vi "Simple UDP - Receiver.vi"() -> ()   [LabVIEW 2014]
doc: "The UDP protocol differs from TCP in that there is no error-checking with the packets of information that are sent, and thus no guarantee whatsoever that an intended recipient will actually receive a given piece of data.\n\nUDP does offer the ability to \"broadcast\" data across a network--simply specify an IP Address of all ones (255.255.255.255) to attempt to broadcast information network-wide. Keep in mind that routers and other network hardware will generally refuse to forward the broadcast beyond certain points, so the extent of the broadcast will in practice be limited."
panel:
  out "Waveform Chart":u8(graph)
  in  "Stop":bool
  # "Overview: Demonstrates the use of the UDP functions to receive data over a UDP connection.\nInstructions:\n1. Ensure Simple UDP - Sender.vi is already running.\n2. Run the VI.\n3. Click Stop to stop the VI."
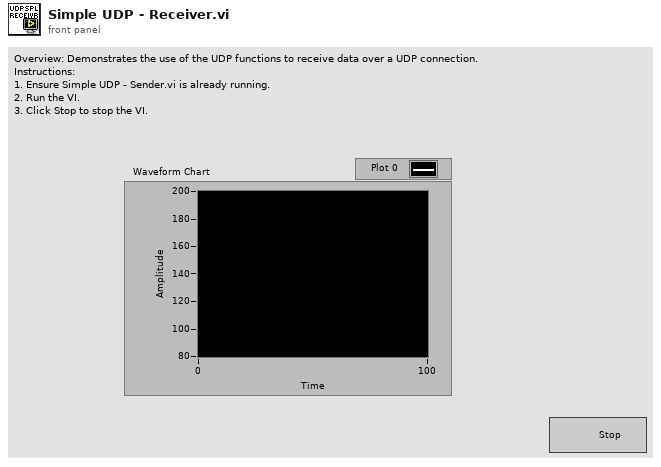
[diagram p1: front panel]
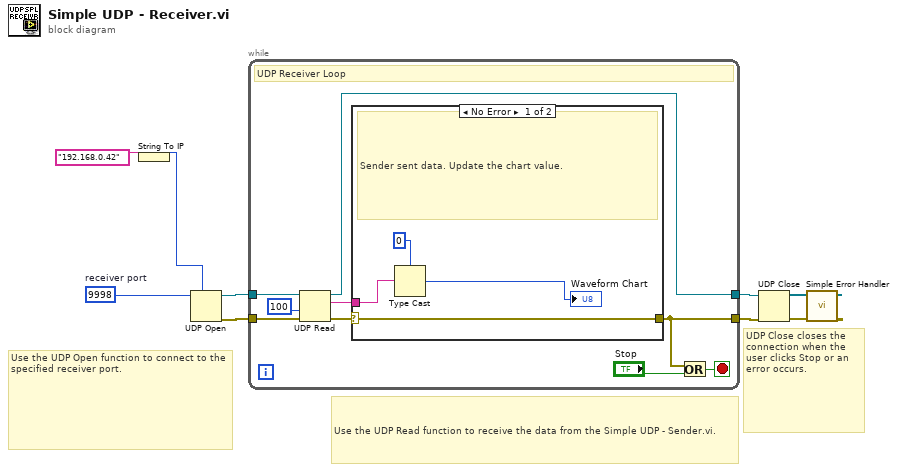
[diagram p0: block diagram]
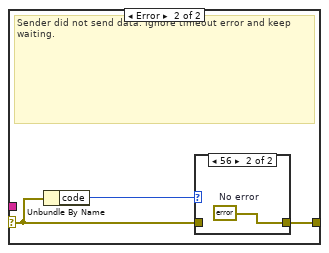
[diagram p2: hidden frame]
diagram:
  w3 = u16 9998  # receiver port
  # "UDP Close closes the connection when the user clicks Stop or an error occurs."
  # "Use the UDP Open function to connect to the specified receiver port."
  # "Use the UDP Read function to receive the data from the Simple UDP - Sender.vi."
  n1 = String To IP(1:"192.168.0.42" ("name")) -> (0:w1:u32)
  n2 = UDP Open(7:w1, 11:w3) -> (port=w4:refnum<k16>, 0:w5:errorcluster)  [unwired: 3 in, 1 out]
  n3 = while {
    tunnel: w4 -> [w17]
    tunnel: [w9] -> w8
    tunnel: w5 -> [w14]
    tunnel: [w10] -> w6
    stop <- w15 stop-if-true
    # "UDP Receiver Loop"
    n4 = UDP Read(connection ID=w17, timeout ms (25000)=100, 8:w14) -> (data out=w12:string, error out=w11:errorcluster, 3:w9:refnum<k16>)  [unwired: 3 out]
    n5 = case shown="No Error" w11 {
      selector: w11 -> [w21 w23]
      tunnel: w12 -> [w20 _]
      tunnel: [w21 w22] -> w10
      frame No Error {
        # "Sender sent data. Update the chart value."
        n6 = Type Cast(type=u8 0 ("timeout ms (25000)"), x=w20) -> (*(type *) &x=→"Waveform Chart":u8)
      }
      frame Error {
        # "Sender did not send data. Ignore timeout error and keep waiting."
        n7 = Unbundle By Name(w23) -> ("code"=w24:i32)
        n8 = case shown="56" w24 {
          tunnel: w23 -> [w25 _]
          tunnel: [w25 w26] -> w22
          frame Default {
          }
          frame 56 {
            w26 = errorcluster {"status"=FALSE, "code"=0, "source"=""}  # No error
          }
        }
      }
    }
    n9 = Or(x=w10, y="Stop") -> (x .or. y?=w15:bool)
  }
  n10 = UDP Close(connection ID=w8, 8:w6) -> (error out=w7:errorcluster)  [unwired: 1 out]
  n11 = call <vilib>:"Simple Error Handler.vi"("error in (no error)"=w7) -> ()  [unwired: 1 in, 8 out]
